vi "MVC Collect File Check.vi"(8 "error in (no error)":errorcluster, 10 "GUI helper Q":refnum<queue>, 11 "GUI in":refnum<class "GUI.lvclass">) -> (0 "error out":errorcluster, 3 "GUI out":refnum<class "GUI.lvclass">)   [LabVIEW 2020, in "GUI.lvlib" / "GUI.lvclass"]
uses:
  GUI.lvclass
  Task Active Enum df.ctl
  GUI.lvclass/GUI.ctl
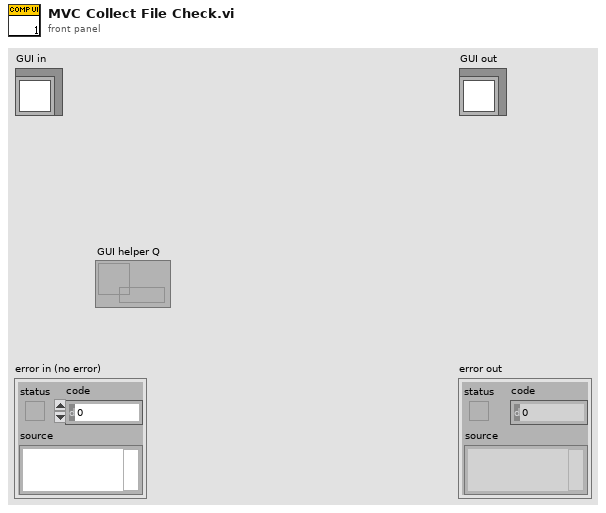
[diagram p1: front panel]
types:
  T1 = typedef "Task Active Enum df.ctl" = enum16{"Idle", "Start Freq Task", "Start Freq Task and Accel", "Start Scanning Task", "Start Scanning Task and Accel", "Preview Template", "Collect MVC", "Calibrate Force", "Calibrate Potentiometers", "Stop Helper"}
  T2 = typedef "Subject and File df.ctl" = cluster{"File Save Path":path, "File Name ":string}
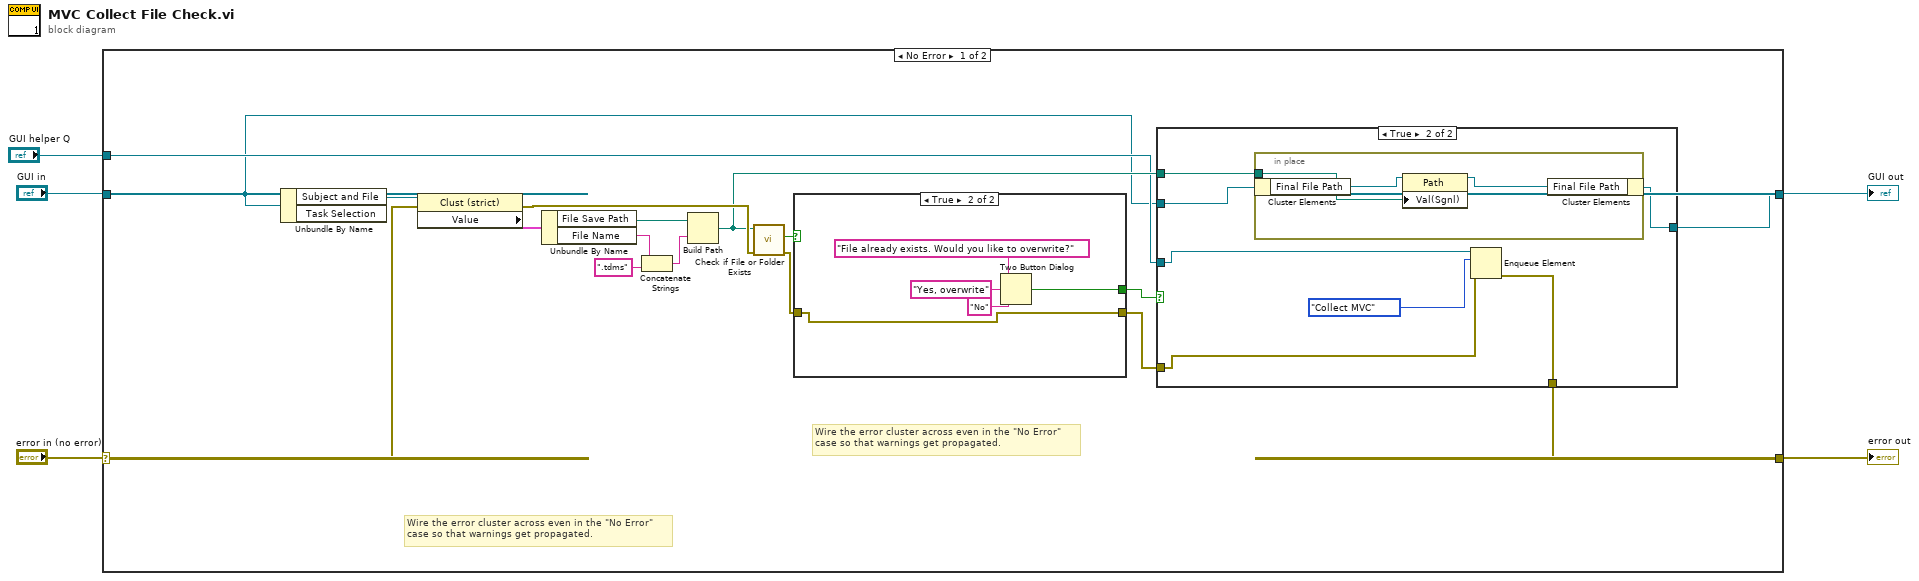
[diagram p0: block diagram]
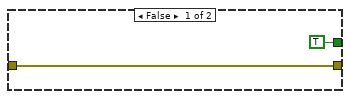
[diagram p3: hidden frame]
diagram:
  n1 = case shown="No Error" "error in (no error)" {
    selector: "error in (no error)" -> [w6 w43]
    tunnel: [w7 w43] -> w4
    tunnel: [w8 w42] -> w2
    tunnel: "GUI in" -> [w9 w42]
    tunnel: "GUI helper Q" -> [w10 _]
    frame No Error {
      # "Wire the error cluster across even in the \"No Error\"\ncase so that warnings get propagated."
      # "Wire the error cluster across even in the \"No Error\"\ncase so that warnings get propagated."
      n2 = Unbundle By Name(w9) -> ("Subject and File"=w22:refnum<vi>)  [unwired: 1 out]
      n3 = property class="Clust (strict)"(reference=w22, error in=w6) -> (error out=w16:errorcluster, "Value"=w21:T2)  [unwired: 1 out]
      n4 = Unbundle By Name(w21) -> ("File Save Path"=w20:path, "File Name"=w19:string)
      n5 = Concatenate Strings(w19, ".tdms" ("string")) -> (w17:string)
      n6 = Build Path(base path=w20, name or relative path=w17) -> (appended path=w11:path)
      n7 = call <vilib>:"Check if File or Folder Exists.vi"("error in (no error)"=w16, "path"=w11) -> ("error out"=w13:errorcluster, "file or folder exists?"=w15:bool)  [unwired: 7 in, 1 out]
      n8 = case shown="True" w15 {
        tunnel: [TRUE ("T button?") w38] -> w14
        tunnel: w13 -> [w35 w37]
        tunnel: [w35 w37] -> w12
        frame False {
        }
        frame True {
          n9 = Two Button Dialog(message="File already exists. Would you like to overwrite?", 1:"No" ("F button name (\"Cancel\")"), 2:"Yes, overwrite" ("T button name (\"OK\")")) -> (T button?=w38:bool)
        }
      }
      n10 = case shown="True" w14 {
        tunnel: w12 -> [w23 w26]
        tunnel: [w23 w25] -> w7
        tunnel: w9 -> [w24 w31]
        tunnel: [w24 w30] -> w8
        tunnel: w11 -> [_ w29]
        tunnel: w10 -> [_ w27]
        frame False {
        }
        frame True {
          n11 = in-place {
            in-place-border: w29 -> [w32]
            n12 = in-place-cluster #1(w31) -> ("Final File Path"=w34:refnum<vi>)
            n13 = property class="Path"(reference=w34, "Val(Sgnl)"=w32) -> (reference out=w33:refnum<vi>)  [unwired: 1 in, 1 out]
            n14 = in-place-cluster #1("Final File Path"=w33) -> (w30:refnum<class "GUI.lvclass">)
          }
          n15 = Enqueue Element(queue=w27, element=Task_Active_Enum_df."Collect MVC", error in (no error)=w26) -> (error out=w25:errorcluster)  [unwired: 1 in, 2 out]
        }
      }
    }
    frame Error {
    }
  }
  "error out" <- w4
  "GUI out" <- w2
